vi "Insert_Wires.vi"(10 "Terminal Map Out":map{string, T3}(c390), 11 "cluster in":T1) -> (3 "output cluster":T1)   [LabVIEW 2025]
uses:
  Terminal.ctl
  bd.ctl
  Classes/Node/Node.lvclass
  wire.ctl
  <vilib>/Utility/error.llb/DialogType.ctl
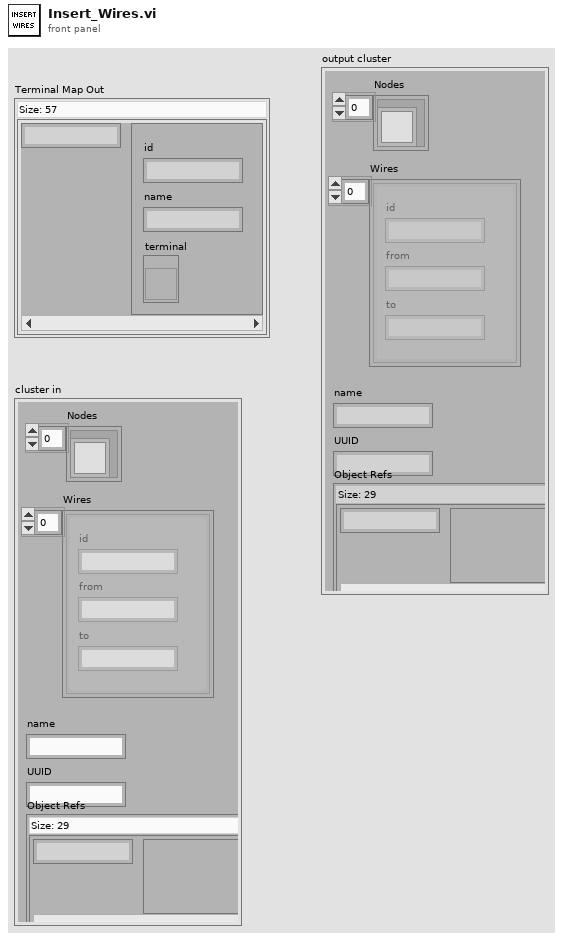
[diagram p1: front panel]
types:
  T1 = typedef "bd.ctl" = cluster{"Nodes":refnum<class "Node.lvclass">[], "Wires":T2[], "name":string, "UUID":string, "Object Refs":map{string, variant}}
  T2 = typedef "wire.ctl" = cluster{"id":string, "from":string, "to":string}
  T3 = typedef "Terminal.ctl" = cluster{"id":string, "name":string, "terminal":refnum<vi>}
  T4 = typedef "DialogType.ctl" = u16
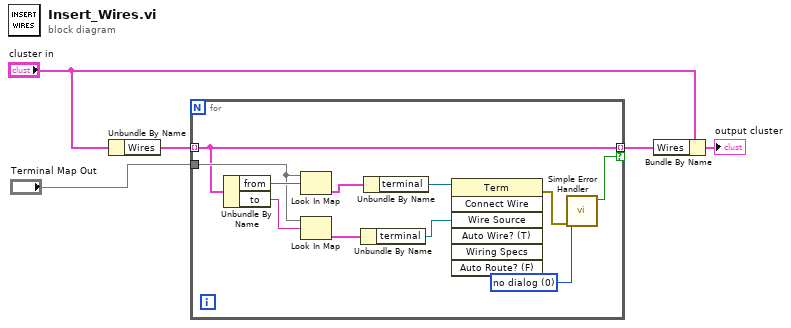
[diagram p0: block diagram]
diagram:
  n1 = Unbundle By Name("cluster in") -> ("Wires"=w4:T2[])
  n2 = for {
    tunnel: w4 -> [w9] mode=indexing
    tunnel: "Terminal Map Out" -> [w15]
    tunnel: [w9] -> w3 mode=indexing if=w6
    w7 = T4 0 items=["no dialog", "OK message", "continue or stop message", "OK message + warnings", "continue/stop + warnings"] ("type of dialog (OK msg:1)")
    n3 = Unbundle By Name(w9) -> ("from"=w16:string, "to"=w14:string)
    n4 = Look In Map(map=w15, key=w16) -> (value=w13:T3)  [unwired: 1 in, 1 out]
    n5 = Look In Map(map=w15, key=w14) -> (value=w12:T3)  [unwired: 1 in, 1 out]
    n6 = Unbundle By Name(w12) -> ("terminal"=w10:refnum<vi>)
    n7 = Unbundle By Name(w13) -> ("terminal"=w11:refnum<vi>)
    n8 = invoke class="Term" method="Connect Wire"(reference=w11, "Wire Source"=w10) -> (error out=w8:errorcluster)  [unwired: 5 in, 6 out]
    n9 = call <vilib>:"Simple Error Handler.vi"("type of dialog (OK msg:1)"=w7, "error in (no error)"=w8) -> ("error?"=w6:bool)  [unwired: 3 in, 4 out]
  }
  n10 = Bundle By Name(cluster="cluster in", "Wires"=w3) -> (→"output cluster":T1)
